vi "U32toRgba_1D.vi"(11 "U32":u32[](array[numeric])) -> (3 "Rgba":T1[](array[typedef]))   [LabVIEW 2024, in "OpenLvVision_Image.lvlib" / "DataAccess.lvlib"]
doc: "Convert an number into an cluster"
uses:
  DataAccess.lvlib
  TypeDef/RgbaU32.ctl
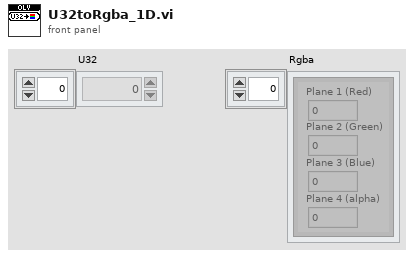
[diagram p1: front panel]
types:
  T1 = typedef "OpenLvVision_Image.lvlib/DataAccess.lvlib/RgbaU32.ctl" = cluster{"Plane 1 (Red)":u8, "Plane 2 (Green)":u8, "Plane 3 (Blue)":u8, "Plane 4 (alpha)":u8}
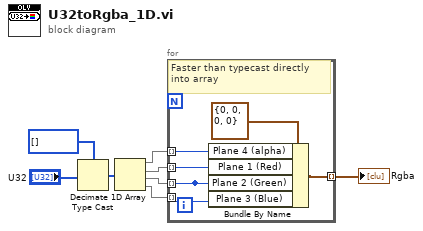
[diagram p0: block diagram]
diagram:
  n1 = Type Cast(type=u8[] [], x="U32") -> (*(type *) &x=w6:u8[])
  n2 = Decimate 1D Array(w6) -> (w5:u8[], w3:u8[], w1:u8[], w4:u8[])
  n3 = for {
    tunnel: w5 -> [w14] mode=indexing
    tunnel: w3 -> [w13] mode=indexing
    tunnel: [w9] -> _ mode=indexing
    tunnel: w4 -> [w12] mode=indexing
    tunnel: [w11] -> w2 mode=indexing
    tunnel: w1 -> [w9] mode=indexing
    # "Faster than typecast directly into array"
    n4 = Bundle By Name(cluster=T1 {"Plane 1 (Red)"=0, "Plane 2 (Green)"=0, "Plane 3 (Blue)"=0, "Plane 4 (alpha)"=0} ("Color"), "Plane 4 (alpha)"=w14, "Plane 1 (Red)"=w13, "Plane 2 (Green)"=w9, "Plane 3 (Blue)"=w12) -> (w11:T1)
  }
  "Rgba" <- w2
